vi "Build Parameter Assignment Array.vi"(8 "error in (no error)":errorcluster, 9 "ParamTypes":string[](array[string]), 10 "ParamValues":string[](array[string]), 11 "ParamNames":string[](array[string])) -> (0 "error out":errorcluster, 2 "Sequence Parameter Assignment refs":T1[](array[typedef]))   [LabVIEW 2015, in "RTSequenceVIs.lvlib"]
uses:
  RTSequenceVIs.lvlib
  <vilib>/NI Veristand/Execution/SequenceExecutionInterface/Sequence Input Assignment Ref.ctl
  NationalInstruments.VeriStand.ClientAPI
  <vilib>/NI Veristand/Execution/SequenceExecutionInterface/Create Sequence Parameter Assignment (Channel).vi
  <vilib>/NI Veristand/Execution/SequenceExecutionInterface/Create Sequence Parameter Assignment (Boolean).vi
  <vilib>/NI Veristand/Execution/SequenceExecutionInterface/Create Sequence Parameter Assignment (Boolean Array).vi
  <vilib>/NI Veristand/Execution/SequenceExecutionInterface/Create Sequence Parameter Assignment (Double).vi
  <vilib>/NI Veristand/Execution/SequenceExecutionInterface/Create Sequence Parameter Assignment (Double Array).vi
  <vilib>/NI Veristand/Execution/SequenceExecutionInterface/Create Sequence Parameter Assignment (I32).vi
  <vilib>/NI Veristand/Execution/SequenceExecutionInterface/Create Sequence Parameter Assignment (I32 Array).vi
  <vilib>/NI Veristand/Execution/SequenceExecutionInterface/Create Sequence Parameter Assignment (I64).vi
  <vilib>/NI Veristand/Execution/SequenceExecutionInterface/Create Sequence Parameter Assignment (I64 Array).vi
  <vilib>/NI Veristand/Execution/SequenceExecutionInterface/Create Sequence Parameter Assignment (U32).vi
  <vilib>/NI Veristand/Execution/SequenceExecutionInterface/Create Sequence Parameter Assignment (U32 Array).vi
  <vilib>/NI Veristand/Execution/SequenceExecutionInterface/Create Sequence Parameter Assignment (U64).vi
  <vilib>/NI Veristand/Execution/SequenceExecutionInterface/Create Sequence Parameter Assignment (U64 Array).vi
  <vilib>/NI Veristand/Execution/SequenceExecutionInterface/NI_VS Sequence Execution Interface.lvlib
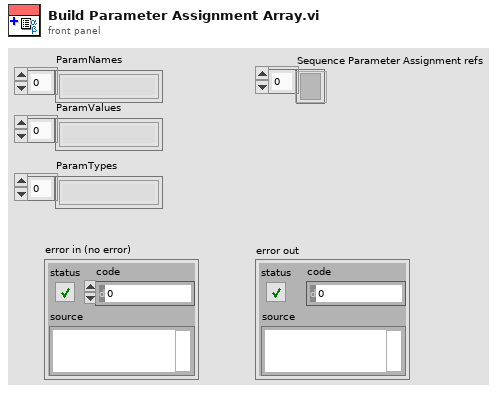
[diagram p1: front panel]
types:
  T1 = typedef "NI_VS Sequence Execution Interface.lvlib/Sequence Input Assignment Ref.ctl" = refnum<k24>
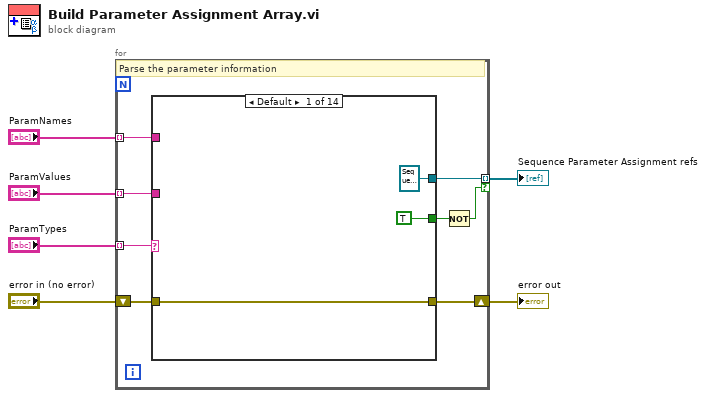
[diagram p0: block diagram]
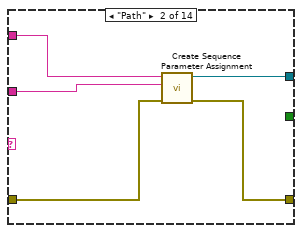
[diagram p2: hidden frame]
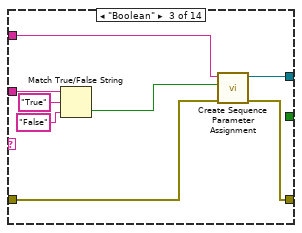
[diagram p3: hidden frame]
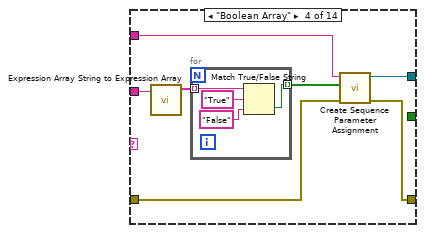
[diagram p4: hidden frame]
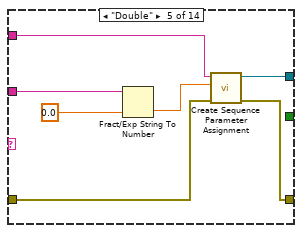
[diagram p5: hidden frame]
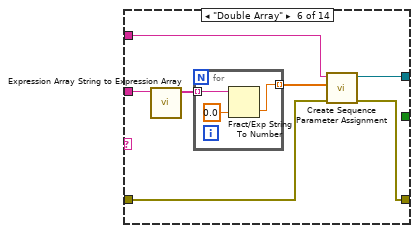
[diagram p6: hidden frame]
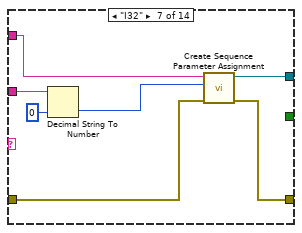
[diagram p7: hidden frame]
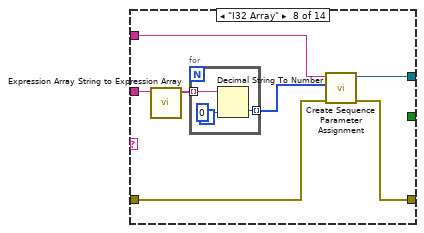
[diagram p8: hidden frame]
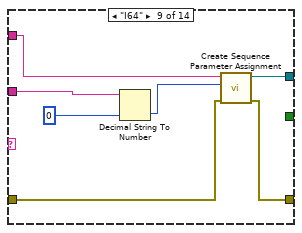
[diagram p9: hidden frame]
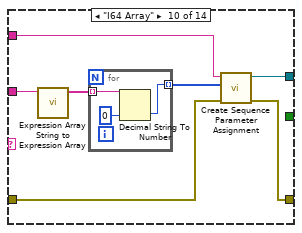
[diagram p10: hidden frame]
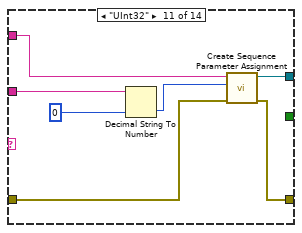
[diagram p11: hidden frame]
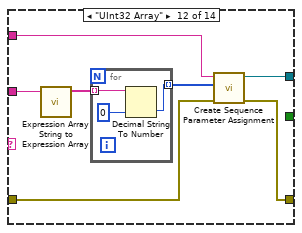
[diagram p12: hidden frame]
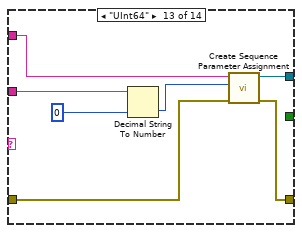
[diagram p13: hidden frame]
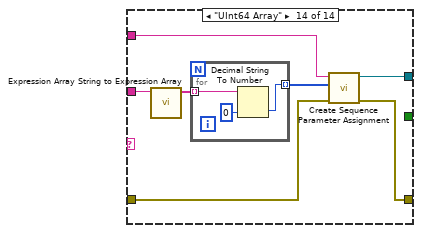
[diagram p14: hidden frame]
diagram:
  n1 = for {
    tunnel: "ParamTypes" -> [w14] mode=indexing
    tunnel: "ParamValues" -> [w13] mode=indexing
    tunnel: "ParamNames" -> [w12] mode=indexing
    shift-right: [w10] -> w2
    shift-left: "error in (no error)" -> [w11]
    tunnel: [w9] -> w3 mode=indexing if=w7
    # "Parse the parameter information"
    n2 = case shown="Default" w14 {
      tunnel: w13 -> [_ w18 w29 w33 w46 w51 w65 w67 w79 w84 w95 w101 w113 w118]
      tunnel: w12 -> [_ w22 w30 w37 w48 w55 w61 w70 w80 w88 w96 w104 w114 w122]
      tunnel: w11 -> [w16 w21 w25 w36 w44 w54 w63 w72 w78 w87 w94 w103 w111 w120]
      tunnel: [w16 w20 w24 w35 w43 w53 w60 w69 w77 w86 w93 w102 w110 w119] -> w10
      tunnel: [T1 refnum ("Sequence Parameter Assignment Ref") w19 w23 w34 w42 w52 w59 w68 w76 w85 w97 w105 w112 w121] -> w9
      tunnel: [TRUE _ _ _ _ _ _ _ _ _ _ _ _ _] -> w8
      frame Default {
      }
      frame "Path" {
        n3 = call-poly <vilib>:"Create Sequence Parameter Assignment.vi"("error in (no error)"=w21, "Channel"=w18, "Parameter Name"=w22) -> ("error out"=w20:errorcluster, "Sequence Parameter Assignment Ref"=w19:T1)  [unwired: 7 in]
      }
      frame "Boolean" {
        n4 = Match True/False String(2:"False" ("false string"), 3:"True" ("true string"), 4:w29) -> (0:w26:bool)  [unwired: 1 out]
        n5 = call-poly <vilib>:"Create Sequence Parameter Assignment.vi"("error in (no error)"=w25, "Value"=w26, "Parameter Name"=w30) -> ("error out"=w24:errorcluster, "Sequence Parameter Assignment Ref"=w23:T1)  [unwired: 7 in]
      }
      frame "Boolean Array" {
        n6 = call "Expression Array String to Expression Array.vi"("Expression Array String"=w33) -> ("Expression Array"=w32:string[])  [unwired: 10 in]
        n7 = for {
          tunnel: w32 -> [w39] mode=indexing
          tunnel: [w38] -> w31 mode=indexing
          n8 = Match True/False String(2:"False" ("false string"), 3:"True" ("true string"), 4:w39) -> (0:w38:bool)  [unwired: 1 out]
        }
        n9 = call-poly <vilib>:"Create Sequence Parameter Assignment.vi"("error in (no error)"=w36, "Value"=w31, "Parameter Name"=w37) -> ("error out"=w35:errorcluster, "Sequence Parameter Assignment Ref"=w34:T1)  [unwired: 7 in]
      }
      frame "Double" {
        n10 = Fract/Exp String To Number(string=w46, default (0 dbl)=0.0 ("default (0 I32)")) -> (number=w45:dbl)  [unwired: 2 in, 1 out]
        n11 = call-poly <vilib>:"Create Sequence Parameter Assignment.vi"("error in (no error)"=w44, "Value"=w45, "Parameter Name"=w48) -> ("error out"=w43:errorcluster, "Sequence Parameter Assignment Ref"=w42:T1)  [unwired: 7 in]
      }
      frame "Double Array" {
        n12 = call "Expression Array String to Expression Array.vi"("Expression Array String"=w51) -> ("Expression Array"=w50:string[])  [unwired: 10 in]
        n13 = for {
          tunnel: w50 -> [w57] mode=indexing
          tunnel: [w56] -> w49 mode=indexing
          n14 = Fract/Exp String To Number(string=w57, default (0 dbl)=0.0 ("default (0 I32)")) -> (number=w56:dbl)  [unwired: 2 in, 1 out]
        }
        n15 = call-poly <vilib>:"Create Sequence Parameter Assignment.vi"("error in (no error)"=w54, "Value"=w49, "Parameter Name"=w55) -> ("error out"=w53:errorcluster, "Sequence Parameter Assignment Ref"=w52:T1)  [unwired: 7 in]
      }
      frame "I32" {
        n16 = Decimal String To Number(string=w65, default (0L)=0 ("default (0 I32)")) -> (number=w62:i32)  [unwired: 1 in, 1 out]
        n17 = call-poly <vilib>:"Create Sequence Parameter Assignment.vi"("error in (no error)"=w63, "Value"=w62, "Parameter Name"=w61) -> ("error out"=w60:errorcluster, "Sequence Parameter Assignment Ref"=w59:T1)  [unwired: 7 in]
      }
      frame "I32 Array" {
        n18 = call "Expression Array String to Expression Array.vi"("Expression Array String"=w67) -> ("Expression Array"=w66:string[])  [unwired: 10 in]
        n19 = for {
          tunnel: [w74] -> w71 mode=indexing
          tunnel: w66 -> [w73] mode=indexing
          n20 = Decimal String To Number(string=w73, default (0L)=0 ("default (0 I32)")) -> (number=w74:i32)  [unwired: 1 in, 1 out]
        }
        n21 = call-poly <vilib>:"Create Sequence Parameter Assignment.vi"("error in (no error)"=w72, "Value"=w71, "Parameter Name"=w70) -> ("error out"=w69:errorcluster, "Sequence Parameter Assignment Ref"=w68:T1)  [unwired: 7 in]
      }
      frame "I64" {
        n22 = Decimal String To Number(string=w79, default (0L)=i64 0 ("default (0 I32)")) -> (number=w81:i64)  [unwired: 1 in, 1 out]
        n23 = call-poly <vilib>:"Create Sequence Parameter Assignment.vi"("error in (no error)"=w78, "Value"=w81, "Parameter Name"=w80) -> ("error out"=w77:errorcluster, "Sequence Parameter Assignment Ref"=w76:T1)  [unwired: 7 in]
      }
      frame "I64 Array" {
        n24 = call "Expression Array String to Expression Array.vi"("Expression Array String"=w84) -> ("Expression Array"=w83:string[])  [unwired: 10 in]
        n25 = for {
          tunnel: [w91] -> w89 mode=indexing
          tunnel: w83 -> [w90] mode=indexing
          n26 = Decimal String To Number(string=w90, default (0L)=i64 0 ("default (0 I32)")) -> (number=w91:i64)  [unwired: 1 in, 1 out]
        }
        n27 = call-poly <vilib>:"Create Sequence Parameter Assignment.vi"("error in (no error)"=w87, "Value"=w89, "Parameter Name"=w88) -> ("error out"=w86:errorcluster, "Sequence Parameter Assignment Ref"=w85:T1)  [unwired: 7 in]
      }
      frame "UInt32" {
        n28 = Decimal String To Number(string=w95, default (0L)=u32 0 ("default (0 I32)")) -> (number=w98:u32)  [unwired: 1 in, 1 out]
        n29 = call-poly <vilib>:"Create Sequence Parameter Assignment.vi"("error in (no error)"=w94, "Value"=w98, "Parameter Name"=w96) -> ("error out"=w93:errorcluster, "Sequence Parameter Assignment Ref"=w97:T1)  [unwired: 7 in]
      }
      frame "UInt32 Array" {
        n30 = call "Expression Array String to Expression Array.vi"("Expression Array String"=w101) -> ("Expression Array"=w100:string[])  [unwired: 10 in]
        n31 = for {
          tunnel: [w108] -> w106 mode=indexing
          tunnel: w100 -> [w107] mode=indexing
          n32 = Decimal String To Number(string=w107, default (0L)=u32 0 ("default (0 I32)")) -> (number=w108:u32)  [unwired: 1 in, 1 out]
        }
        n33 = call-poly <vilib>:"Create Sequence Parameter Assignment.vi"("error in (no error)"=w103, "Value"=w106, "Parameter Name"=w104) -> ("error out"=w102:errorcluster, "Sequence Parameter Assignment Ref"=w105:T1)  [unwired: 7 in]
      }
      frame "UInt64" {
        n34 = Decimal String To Number(string=w113, default (0L)=u64 0 ("default (0 I32)")) -> (number=w115:u64)  [unwired: 1 in, 1 out]
        n35 = call-poly <vilib>:"Create Sequence Parameter Assignment.vi"("error in (no error)"=w111, "Value"=w115, "Parameter Name"=w114) -> ("error out"=w110:errorcluster, "Sequence Parameter Assignment Ref"=w112:T1)  [unwired: 7 in]
      }
      frame "UInt64 Array" {
        n36 = call "Expression Array String to Expression Array.vi"("Expression Array String"=w118) -> ("Expression Array"=w117:string[])  [unwired: 10 in]
        n37 = for {
          tunnel: [w125] -> w123 mode=indexing
          tunnel: w117 -> [w124] mode=indexing
          n38 = Decimal String To Number(string=w124, default (0L)=u64 0 ("default (0 I32)")) -> (number=w125:u64)  [unwired: 1 in, 1 out]
        }
        n39 = call-poly <vilib>:"Create Sequence Parameter Assignment.vi"("error in (no error)"=w120, "Value"=w123, "Parameter Name"=w122) -> ("error out"=w119:errorcluster, "Sequence Parameter Assignment Ref"=w121:T1)  [unwired: 7 in]
      }
    }
    n40 = Not(x=w8) -> (.not. x?=w7:bool)
  }
  "Sequence Parameter Assignment refs" <- w3
  "error out" <- w2
